vi "will_waypoints_hit_obstacles.vi"(0 "Obstacle array":refnum<class "Obstacle.lvclass">[](array[class]), 1 "WP array":refnum<class "Waypoint.lvclass">[](array[class]), 2 "Boat Location":T1 {"North" format="%#_10f"; "East" format="%#_8f"}) -> (7 "Will boat hit any obstacles?":bool)   [LabVIEW 2013]
doc: "Checks whether an array of waypoints will hit the obstacle array.\n\nEric Schneider, September 2014"
uses:
  Obstacle.lvclass
  Data/TypeDefs/UTM Location.ctl
  Waypoint/Waypoint.lvclass
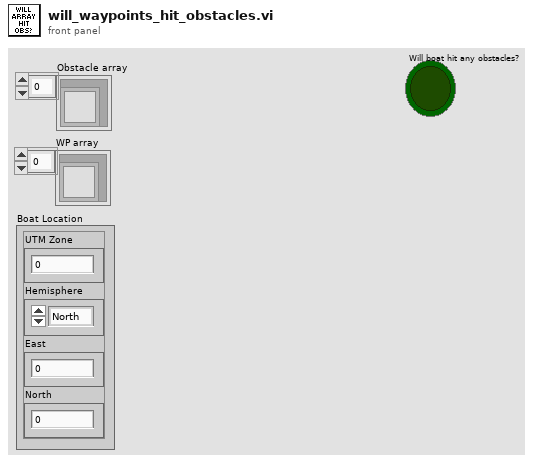
[diagram p1: front panel]
types:
  T1 = typedef "UTM Location.ctl" = cluster{"UTM Zone":dbl, "Hemisphere":enum16{"North", "South"}, "East":dbl, "North":dbl}
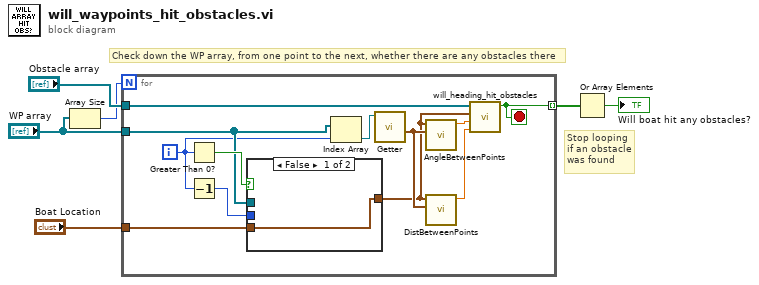
[diagram p0: block diagram]
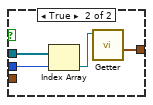
[diagram p2: hidden frame]
diagram:
  # "Stop looping if an obstacle was found"
  # "Check down the WP array, from one point to the next, whether there are any obstacles there"
  n1 = Array Size(array="WP array") -> (size(s)=w1:i32)
  n2 = for {
    N: w1 -> [_]
    tunnel: "Obstacle array" -> [w18]
    tunnel: [w8] -> w6 mode=indexing
    tunnel: "WP array" -> [w13]
    tunnel: "Boat Location" -> [w15]
    i -> [w7]
    stop <- w8 stop-if-true
    n3 = Greater Than 0?(x=w7) -> (x > 0?=w17:bool)
    n4 = Decrement(x=w7) -> (x-1=w16:i32)
    n5 = case shown="False" w17 {
      tunnel: w13 -> [_ w23]
      tunnel: w16 -> [_ w22]
      tunnel: [w19 w20] -> w11
      tunnel: w15 -> [w19 _]
      frame False {
      }
      frame True {
        n6 = Index Array(array=w23, index=w22) -> (element=w21:refnum<class "Waypoint.lvclass">)
        n7 = call "Getter.vi"("Waypoint In"=w21) -> ("Coords"=w20:T1)  [unwired: 6 in, 4 out]
      }
    }
    n8 = Index Array(array=w13, index=w7) -> (element=w14:refnum<class "Waypoint.lvclass">)
    n9 = call "Getter.vi"("Waypoint In"=w14) -> ("Coords"=w12:T1)  [unwired: 6 in, 4 out]
    n10 = call "AngleBetweenPoints.vi"("Point 2"=w12, "Point 1"=w11) -> ("Angle from P1 to P2"=w9:dbl)  [unwired: 9 in]
    n11 = call "DistBetweenPoints.vi"("UTM Location 2"=w12, "UTM Location 1"=w11) -> ("Distance from 1 to 2"=w10:dbl)  [unwired: 9 in]
    n12 = call "will_heading_hit_obstacles.vi"("Distance to check (m)"=w10, "Heading"=w9, "Boat Location"=w11, "Obstacle array"=w18) -> ("Will boat hit any obstacles?"=w8:bool)  [unwired: 7 in]
  }
  n13 = Or Array Elements(Boolean array=w6) -> (logical OR=→"Will boat hit any obstacles?":bool)
